vi "EnqueueCommand.vi"(6 "cmdData":string, 7 "Priority?(F)":bool, 8 "error in (no error)":errorcluster, 9 "data":string, 10 "command":string, 11 "Data Cluster":T1) -> (0 "error out":errorcluster)   [LabVIEW 2015, in "ISA010_module.lvlib"]
uses:
  ISA010_module.lvlib
  Module Data--cluster.ctl
  ISA010/ISA010.lvclass
  libraries/ModBUS.lvlibp/Base/Modbus.lvclass
  ISA010/Command.ctl
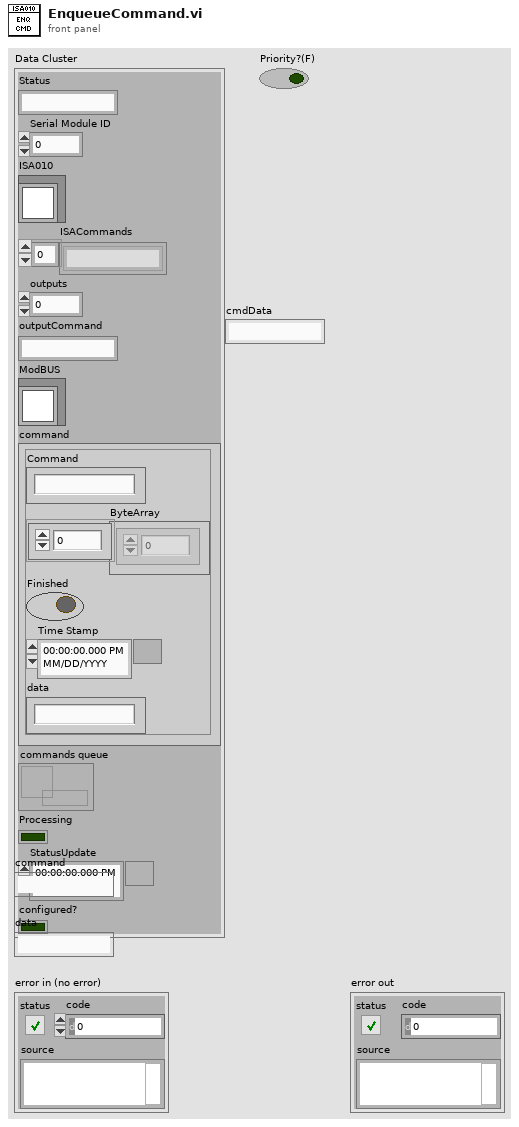
[diagram p1: front panel]
types:
  T1 = typedef "ISA010_module.lvlib/Module Data--cluster.ctl" = cluster{"Status":string, "Serial Module ID":i32, "ISA010":refnum<class "ISA010.lvclass">, "ISACommands":string[], "outputs":u16, "outputCommand":string, "ModBUS":refnum<class "Modbus.lvclass">, "command":T2, "commands queue":refnum<queue>, "Processing":bool, "StatusUpdate":timestamp, "configured?":bool}
  T2 = typedef "Command.ctl" = cluster{"Command":string, "ByteArray":u8[], "Finished":bool, "Time Stamp":timestamp, "data":string}
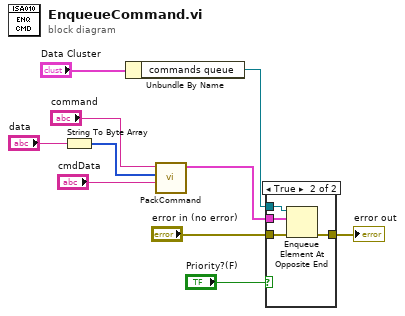
[diagram p0: block diagram]
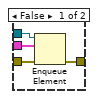
[diagram p2: hidden frame]
diagram:
  n1 = String To Byte Array(string="data") -> (unsigned byte array=w5:u8[])
  n2 = Unbundle By Name("Data Cluster") -> ("commands queue"=w9:refnum<queue>)
  n3 = call "PackCommand.vi"("data"="cmdData", "unsigned byte array"=w5, "ISACommand"="command") -> ("command"=w6:T2)  [unwired: 8 in]
  n4 = case shown="True" "Priority?(F)" {
    tunnel: w9 -> [w14 w15]
    tunnel: [w13 w17] -> w8
    tunnel: "error in (no error)" -> [w12 w18]
    tunnel: w6 -> [w11 w16]
    frame False {
      n5 = Enqueue Element(queue=w14, element=w11, error in (no error)=w12) -> (error out=w13:errorcluster)  [unwired: 1 in, 2 out]
    }
    frame True {
      n6 = Enqueue Element At Opposite End(queue=w15, element=w16, error in (no error)=w18) -> (error out=w17:errorcluster)  [unwired: 1 in, 2 out]
    }
  }
  "error out" <- w8
